vi "get current index.vi"(8 "error in (no error)":errorcluster, 11 "Group run list in":string[][](array[string])) -> (0 "error out":errorcluster, 2 "current index":i32, 3 "Group run list out":string[][](array[string]))   [LabVIEW 2016]
doc: "This vi determines where in the run order which index is being \nused"
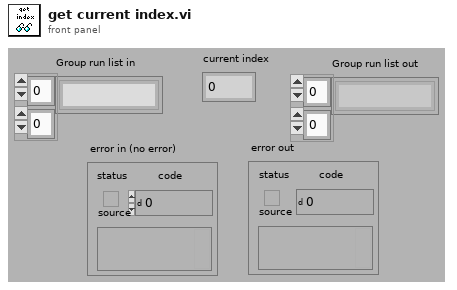
[diagram p1: front panel]
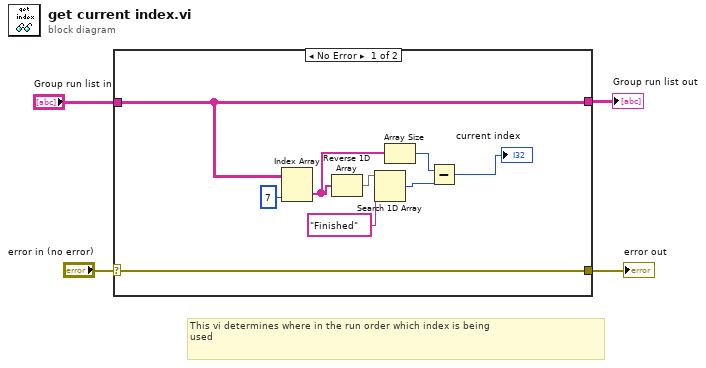
[diagram p0: block diagram]
diagram:
  # "This vi determines where in the run order which index is being \nused"
  n1 = case shown="No Error" "error in (no error)" {
    selector: "error in (no error)" -> [w6 w15]
    tunnel: [w6 w15] -> w3
    tunnel: "Group run list in" -> [w5 w14]
    tunnel: [w5 w14] -> w1
    frame No Error {
      n2 = Index Array(array=w5, index (col)=7 ("disabled index (col)")) -> (element=w10:string[])  [unwired: 1 in]
      n3 = Reverse 1D Array(array=w10) -> (reversed array=w12:string[])
      n4 = Search 1D Array(1D array=w12, element="Finished") -> (index of element=w9:i32)  [unwired: 1 in]
      n5 = Array Size(array=w10) -> (size(s)=w8:i32)
      n6 = Subtract(x=w8, y=w9) -> (x-y=→"current index":i32)
    }
    frame Error {
    }
  }
  "error out" <- w3
  "Group run list out" <- w1
